vi "Reset.vi"(8 "error in (no error)":errorcluster, 10 "Message in":refnum<class "ResetMessage.lvclass">, 11 "RSA in":refnum<class "RSA.lvclass">) -> (0 "error out":errorcluster, 3 "RSA out":refnum<class "RSA.lvclass">)   [LabVIEW 2012, in "RSA.lvclass"]
doc: "The reset method processes the command 'reset'. \n\nResets the internal state of the component (without performing a full initialisation). This could be resetting hardware, or private data to default values."
uses:
  RSA.lvclass
  <vilib>/Distrio/Murmex/ResetMessage/ResetMessage.lvclass
  <vilib>/Distrio/Murmex/Murmex/Murmex.lvclass
  RSA.lvclass/RSA.ctl
panel:
  # "This method is called when the RESET\ntrigger is sent. \n\nOverride this method when your component needs to\nrespond to this trigger. \n\nCall parent for proper implementation"
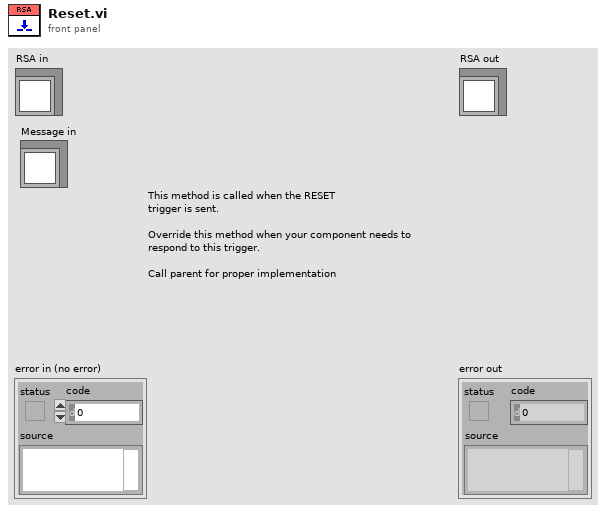
[diagram p1: front panel]
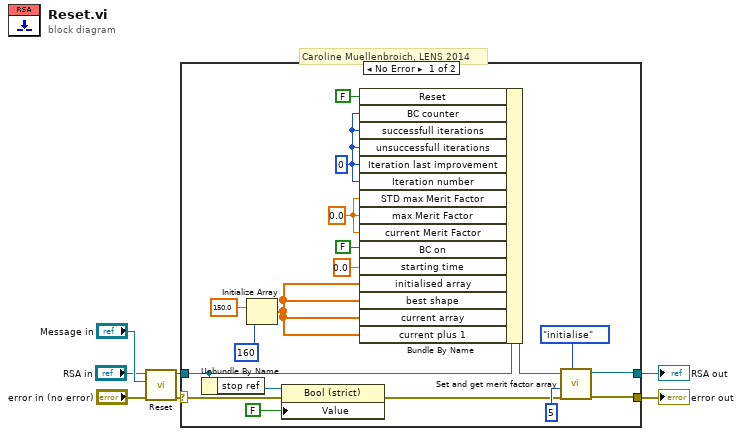
[diagram p0: block diagram]
diagram:
  # "Caroline Muellenbroich, LENS 2014"
  n1 = call-parent "Reset.vi"("error in (no error)"="error in (no error)", "Message in"="Message in", "Murmex in"="RSA in") -> ("error out"=w4:errorcluster, "Murmex out"=w2:refnum<class "RSA.lvclass">)  [unwired: 7 in]
  n2 = case shown="No Error" w4 {
    selector: w4 -> [w9 w26]
    tunnel: [w14 w26] -> w3
    tunnel: w2 -> [w12 w27]
    tunnel: [w15 w27] -> w1
    frame No Error {
      w19 = 0 ("Run time cluster.Iteration number")
      w25 = 0.0 ("Run time cluster.current Merit Factor")
      n3 = Unbundle By Name(w12) -> ("stop ref"=w11:refnum<vi>)
      n4 = Initialize Array(150.0 ("element"), 160 ("dimension size")) -> (w22:dbl[])
      n5 = property class="Bool (strict)"(reference=w11, error in=w9, "Value"=FALSE) -> (error out=w8:errorcluster)  [unwired: 1 out]
      n6 = Bundle By Name(cluster=w12, "Reset"=FALSE ("Run time cluster.Reset"), "BC counter"=w19, "successfull iterations"=w19, "unsuccessfull iterations"=w19, "Iteration last improvement"=w19, "Iteration number"=w19, "STD max Merit Factor"=w25, "max Merit Factor"=w25, "current Merit Factor"=w25, "BC on"=FALSE ("Run time cluster.Timer"), "starting time"=0.0 ("Run time cluster.starting time"), "initialised array"=w22, "best shape"=w22, "current array"=w22, "current plus 1"=w22) -> (w16:refnum<class "RSA.lvclass">)
      n7 = call "Set and get merit factor array.vi"("action"=enum16{"set", "get", "initialise"}."initialise", "error in (no error)"=w8, "array size"=5, "RSA in"=w16) -> ("error out"=w14:errorcluster, "RSA out"=w15:refnum<class "RSA.lvclass">)  [unwired: 4 in, 2 out]
    }
    frame Error {
    }
  }
  "error out" <- w3
  "RSA out" <- w1
